vi "Lvi Thermocouple Channel Settings.vi"(6 "DataFilter":u32, 8 "error in (no error)":errorcluster, 9 "TcType":u32, 10 "Channel":u32, 11 "TaskRef":i32) -> (0 "error out":errorcluster, 2 "function return":u32(ring), 3 "TaskRef out":i32)   [LabVIEW 2022 SP3, in "DtLvLink.lvlib"]
doc: "Calls directly into the entry points of the DLL of the Data Acq SDK to specify the thermocouple type for an analog input task. This VI is used by the higher-level VI, DtOLSetChanThermocoupleOptions."
uses:
  DtLvLink.lvlib
  <userlib>/LV-Link3/DtLvLink_64.dll
panel:
  in  "ReturnCJC":bool
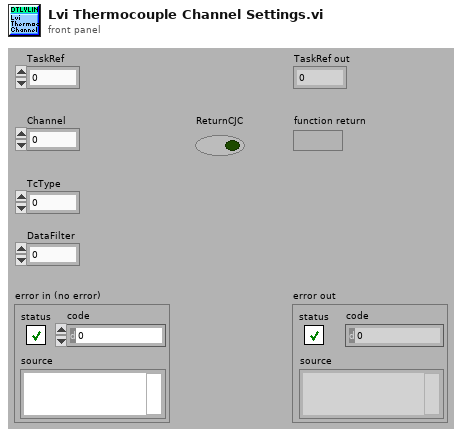
[diagram p1: front panel]
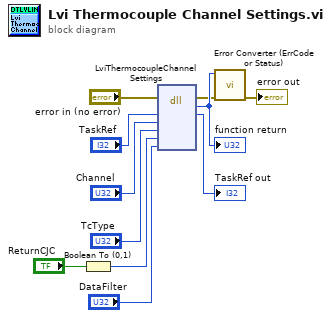
[diagram p0: block diagram]
diagram:
  n1 = Boolean To (0,1)(Boolean="ReturnCJC") -> (0, 1=w5:i16)
  n2 = dll-call lib="C:/Program Files/National Instruments/LabVIEW 2022/user.lib/LV-Link3/DtLvLink_64.*" fn="LviThermocoupleChannelSettings"(error in="error in (no error)", "TaskRef"="TaskRef", "Channel"="Channel", "TcType"="TcType", "ReturnCJC"=w5, "DataFilter"="DataFilter") -> (error out=w3:errorcluster, "return type"=w11:u32, "TaskRef"=→"TaskRef out":i32)  [unwired: 6 in, 1 out]
  "function return" <- w11
  n3 = call "Error Converter (ErrCode or Status).vi"("error in (no error)"=w3, "error code"=w11) -> ("error out"=→"error out":errorcluster)  [unwired: 9 in]
